vi "EventStructureSerial.vi"() -> ()   [LabVIEW 2020]
uses:
  <vilib>/Instr/_visa.llb/VISA Configure Serial Port (Instr).vi
  <vilib>/ErrorRing/Error Ring.xnode
panel:
  in  "Gauge":dbl(knob) scale=0.0..100.0
  in  "Numeric":u16
  in  "VISA resource name":refnum<visa-resource-name>
  in  "Stop Button":bool
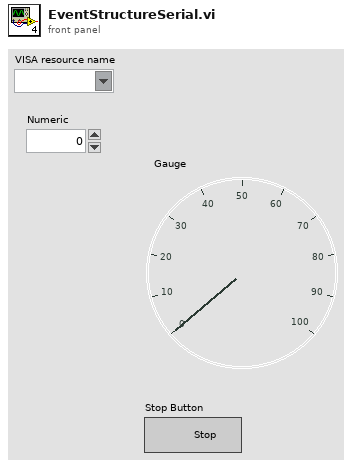
[diagram p1: front panel]
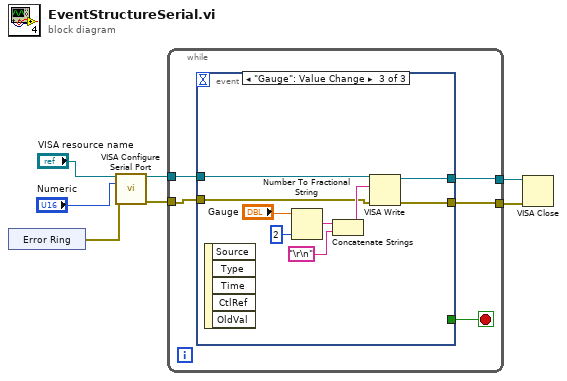
[diagram p0: block diagram]
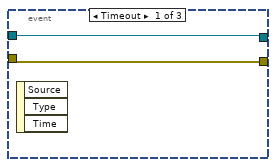
[diagram p2: hidden frame]
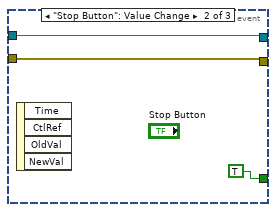
[diagram p3: hidden frame]
diagram:
  n1 = xnode "Error Ring"() -> ("error out"=w5:errorcluster)
  n2 = call-poly "VISA Configure Serial Port"("VISA resource name"="VISA resource name", "baud rate (9600)"="Numeric", "error in (no error)"=w5) -> ("VISA resource name out"=w3:refnum<visa-resource-name>, "error out"=w4:errorcluster)  [unwired: 11 in]
  n3 = while {
    tunnel: w4 -> [w10]
    tunnel: w3 -> [w11]
    tunnel: [w9] -> w2
    tunnel: [w8] -> w1
    stop <- w12 stop-if-true
    n4 = event shown="[2] \"Gauge\": Value Change" {
      selector: _ -> [_ _ _]
      dyn-events: _ -> [_ _ _]
      timeout: _ -> [_ _ _]
      tunnel: [_ TRUE _] -> w12
      tunnel: w11 -> [w14 w16 w21]
      tunnel: w10 -> [w13 w15 w20]
      tunnel: [w14 w16 w19] -> w9
      tunnel: [w13 w15 w18] -> w8
      event Timeout {
        n5 = event-data() -> ()  [unwired: 1 in, 3 out]
      }
      event "Stop Button": Value Change {
        n6 = event-data() -> ()  [unwired: 1 in, 4 out]
      }
      event "Gauge": Value Change {
        n7 = event-data() -> ()  [unwired: 1 in, 5 out]
        n8 = Number To Fractional String(number="Gauge", precision (6)=i16 2) -> (F-format string=w25:string)  [unwired: 2 in]
        n9 = Concatenate Strings(w25, "\r\n") -> (w24:string)
        n10 = VISA Write(VISA resource name=w21, write buffer=w24, error in (no error)=w20) -> (VISA resource name out=w19:refnum<visa-resource-name>, error out=w18:errorcluster)  [unwired: 1 out]
      }
    }
  }
  n11 = VISA Close(VISA resource name=w2, error in (no error)=w1) -> ()  [unwired: 1 out]
